vi "MoveBase.vi"(0 "Speed":dbl min=0.0, 1 "Relative/Absolute\nPosition":enum16{"Relative", "Absolute"}(ring), 2 "connection refnum in":refnum<k5>, 3 "IP address":string, 5 "Speed Units (unit/s)":enum16{"mm", "µm"}(ring), 7 "Target Position":dbl, 9 "Target Position Units":enum16{"mm", "µm"}(ring), 11 "error in":errorcluster, 12 "Axis":enum16{"Z", "Y", "X"}(ring)) -> (4 "approx move time (ms)":i32, 6 "connection refnum out":refnum<k5>, 15 "error out":errorcluster)   [LabVIEW 2023]
doc: "The base function to move the instrument in a chosen direction in a stepwise manner."
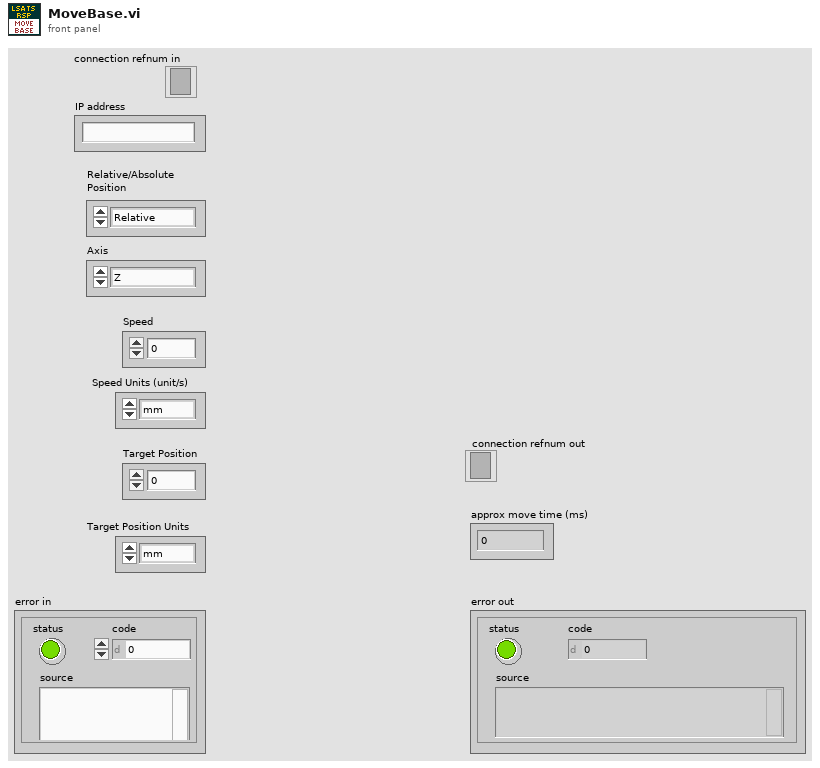
[diagram p1: front panel]
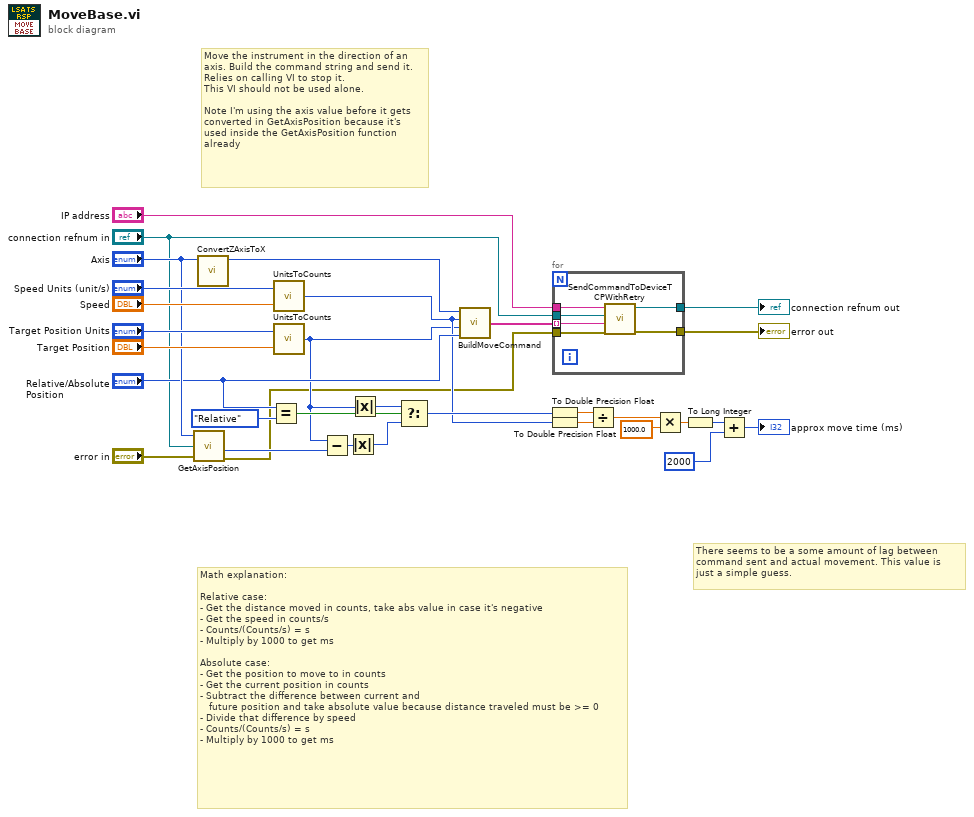
[diagram p0: block diagram]
diagram:
  # "There seems to be a some amount of lag between\ncommand sent and actual movement. This value is\njust a simple guess."
  # "Math explanation:\n\nRelative case:\n- Get the distance moved in counts, take abs value in case it's negative\n- Get the speed in counts/s\n- Counts/(Counts/s) = s\n- Multiply by 1000 to get ms\n\nAbsolute case:\n- Get the position to move to in counts\n- Get the current position in counts\n- Subtract the difference between current and \n   future position and take absolute value because distance traveled must be >= 0\n- Divide that difference by speed\n- Counts/(Counts/s) = s\n- Multiply by 1000 to get ms"
  # "Move the instrument in the direction of an axis. Build the command string and send it. Relies on calling VI to stop it.\nThis VI should not be used alone.\n\nNote I'm using the axis value before it gets converted in GetAxisPosition because it's used inside the GetAxisPosition function already"
  n1 = call "GetAxisPosition.vi"("Axis"="Axis", "connection refnum in"="connection refnum in", "error in"="error in") -> ("numeric result"=w10:i32, "error out"=w1:errorcluster)  [unwired: 2 out]
  n2 = call "ConvertZAxisToX.vi"("Axis in"="Axis") -> ("Axis out"=w25:enum16{"Z", "Y", "X"})  [unwired: 6 in]
  n3 = Equal?(x="Relative/Absolute\nPosition", y=enum16{"Relative", "Absolute"}."Relative") -> (x = y?=w17:bool)
  n4 = call "UnitsToCounts.vi"("Unit Value"="Speed", "Units"="Speed Units (unit/s)") -> ("Counts"=w14:i32)
  n5 = call "UnitsToCounts.vi"("Unit Value"="Target Position", "Units"="Target Position Units") -> ("Counts"=w8:i32)
  n6 = Subtract(x=w8, y=w10) -> (x-y=w21:i32)
  n7 = Absolute Value(x=w21) -> (abs(x)=w16:i32)
  n8 = Absolute Value(x=w8) -> (abs(x)=w9:i32)
  n9 = Select(t=w9, s=w17, f=w16) -> (s? t:f=w15:i32)
  n10 = call "BuildMoveCommand.vi"("Relative/Absolute\nPosition"="Relative/Absolute\nPosition", "Position Counts"=w8, "Speed Counts"=w14, "Axis"=w25) -> ("Command Strings"=w31:string[])
  n11 = To Double Precision Float(number=w15) -> (double precision float=w23:dbl)
  n12 = To Double Precision Float(number=w14) -> (double precision float=w22:dbl)
  n13 = for {
    tunnel: w31 -> [w37] mode=indexing
    tunnel: [w36] -> w24
    tunnel: "IP address" -> [w35]
    tunnel: w1 -> [w34]
    tunnel: "connection refnum in" -> [w33]
    tunnel: [w32] -> w6
    n14 = call "SendCommandToDeviceTCPWithRetry.vi"("error in"=w34, "str command"=w37, "connection refnum in"=w33, "IP address"=w35) -> ("error out"=w36:errorcluster, "connection refnum out"=w32:refnum<k5>)  [unwired: 4 in, 2 out]
  }
  "error out" <- w24
  "connection refnum out" <- w6
  n15 = Divide(x=w23, y=w22) -> (x/y=w13:dbl)
  n16 = Multiply(x=w13, y=1000.0) -> (x*y=w11:dbl)
  n17 = To Long Integer(number=w11) -> (32bit integer=w5:i32)
  n18 = Add(x=w5, y=2000) -> (x+y=→"approx move time (ms)":i32)
